vi "Alpha4.vi"() -> ()   [LabVIEW 2011]
uses:
  <vilib>/vision/NI_Vision_Development_Module.lvlib
panel:
  in  "Threshold Slider":cluster{u8, u8}(slide)={0, 6} scale=0.0..255.0
  in  "Threshold selectoin":bool
  out "Image Enhanced":T1(plugin-control)
  in  "Gamma":sgl(slide)=2.14 scale=0.0..10.0
  in  "Contrast":u8(slide)=60 scale=0.0..255.0
  in  "Brightness":u8(slide)=118 scale=0.0..255.0
  in  "Basic Morphology Operatoin":T2(ring)
  out "Threshold":T1(plugin-control)
  in  "Stop":bool
  in  "Browse":bool
  out "Original Image":T1(plugin-control)
  out "Path to Image":path
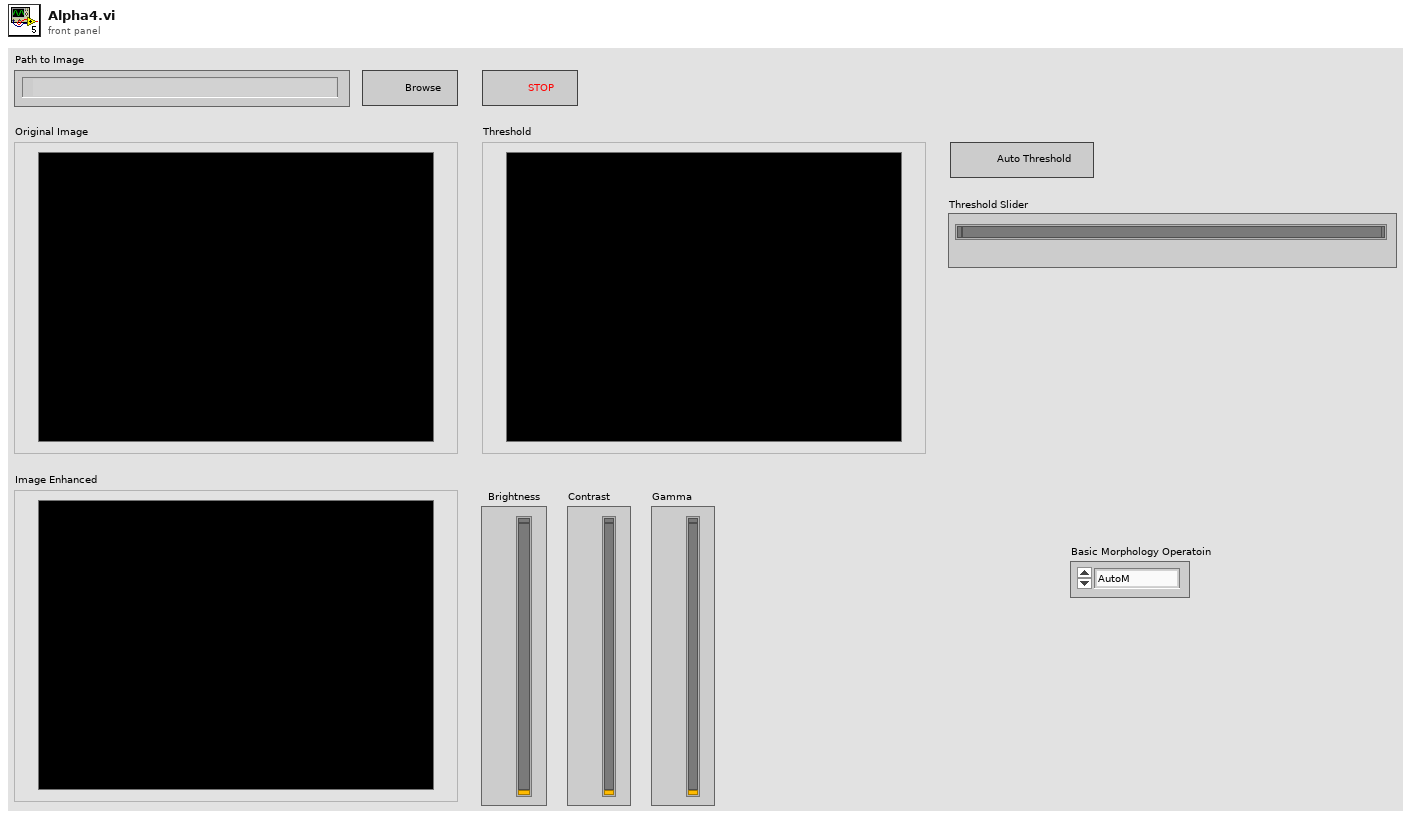
[diagram p1: front panel]
types:
  T1 = typedef "IMAQ Image.ctl" = refnum<image>
  T2 = enum16{"AutoM", "Close", "Dilate", "Erode", "Gradient", "Gradient out", "Gradient in", "Hit miss", "Open", "PClose", "POpen", "Thick", "Thin"}
  T3 = typedef "Image Type" = u32
  T4 = enum8{"Enabled", "Disabled", "Disabled and Grayed Out"}
  T5 = cluster{"Brightness":u8, "Contrast":u8, "Gamma":sgl}
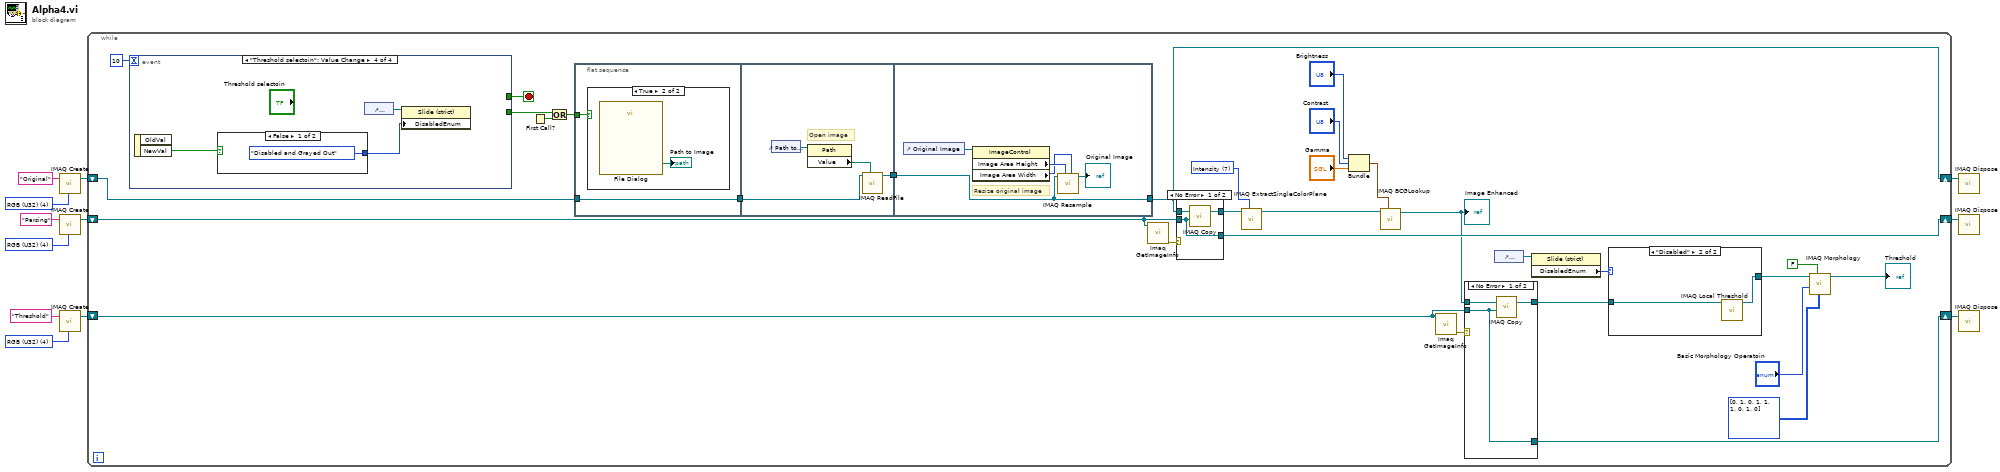
[diagram p0: block diagram]
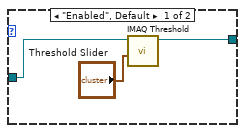
[diagram p2: hidden frame]
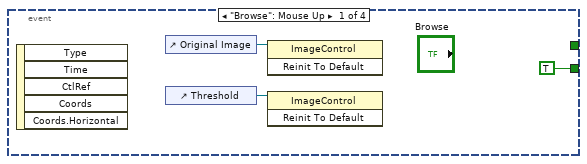
[diagram p6: hidden frame]
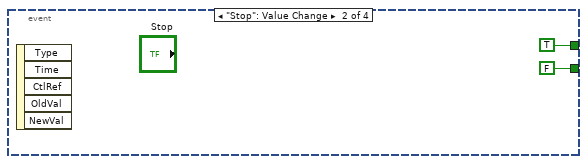
[diagram p7: hidden frame]
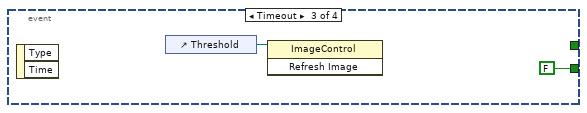
[diagram p8: hidden frame]
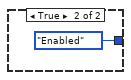
[diagram p9: hidden frame]
diagram:
  w3 = T3 4 items=["Grayscale (U8)", "Grayscale (I16)", "Grayscale (SGL)", "Complex (CSG)", "RGB (U32)", "HSL (U32)", "RGB (U64)", "Grayscale (U16)"] ("Image Type")
  w5 = T3 4 items=["Grayscale (U8)", "Grayscale (I16)", "Grayscale (SGL)", "Complex (CSG)", "RGB (U32)", "HSL (U32)", "RGB (U64)", "Grayscale (U16)"] ("Image Type")
  w8 = T3 4 items=["Grayscale (U8)", "Grayscale (I16)", "Grayscale (SGL)", "Complex (CSG)", "RGB (U32)", "HSL (U32)", "RGB (U64)", "Grayscale (U16)"] ("Image Type")
  n1 = call "IMAQ Create"("Image Name"="Original", "Image Type"=w8) -> ("New Image"=w11:T1)  [unwired: 3 in, 1 out]
  n2 = call "IMAQ Create"("Image Name"="Parsing", "Image Type"=w5) -> ("New Image"=w9:T1)  [unwired: 3 in, 1 out]
  n3 = call "IMAQ Create"("Image Name"="Threshold", "Image Type"=w3) -> ("New Image"=w2:T1)  [unwired: 3 in, 1 out]
  n4 = while {
    shift-right: [w40] -> w7
    shift-left: w11 -> [w35]
    shift-right: [w21] -> w6
    shift-left: w9 -> [w39]
    shift-right: [w18] -> w1
    shift-left: w2 -> [w19]
    stop <- w41 stop-if-true
    w26 = 7 items=["Red", "Green", "Blue", "Hue", "Saturation", "Luminance", "Value", "Intensity"] ("Color Plane")
    n5 = event shown="[3] \"Threshold selectoin\": Value Change" {
      selector: _ -> [_ _ _ _]
      dyn-events: _ -> [_ _ _ _]
      timeout: 10 -> [_ _ _ _]
      tunnel: [_ TRUE _ _] -> w41
      tunnel: [TRUE FALSE FALSE _] -> w38
      event "Browse": Mouse Up {
        n6 = event-data() -> ()  [unwired: 1 in, 5 out]
        n7 = control-ref of="Original Image"() -> (w72:refnum<vi>)
        n8 = control-ref of="Threshold"() -> (w73:refnum<vi>)
        n9 = invoke class="ImageControl" method="Reinit To Default"(reference=w72) -> ()  [unwired: 2 in, 3 out]
        n10 = invoke class="ImageControl" method="Reinit To Default"(reference=w73) -> ()  [unwired: 2 in, 3 out]
      }
      event "Stop": Value Change {
        n11 = event-data() -> ()  [unwired: 1 in, 5 out]
      }
      event Timeout {
        n12 = event-data() -> ()  [unwired: 1 in, 2 out]
        n13 = control-ref of="Threshold"() -> (w77:refnum<vi>)
        n14 = invoke class="ImageControl" method="Refresh Image"(reference=w77) -> ()  [unwired: 2 in, 3 out]
      }
      event "Threshold selectoin": Value Change {
        n15 = event-data() -> ("NewVal"=w79:bool)  [unwired: 1 in, 1 out]
        n16 = case shown="False" w79 {
          tunnel: [T4."Disabled and Grayed Out" ("Disabled") T4."Enabled" ("Disabled")] -> w80
          frame False {
          }
          frame True {
          }
        }
        n17 = control-ref of="Threshold Slider"() -> (w78:refnum<vi>)
        n18 = property class="Slide (strict)"(reference=w78, "DisabledEnum"=w80) -> ()  [unwired: 1 in, 2 out]
      }
    }
    n19 = First Call?() -> (First Call?: T/F=w37:bool)
    n20 = Or(x=w38, y=w37) -> (x .or. y?=w36:bool)
    n21 = flat-sequence {
      tunnel: w36 -> [w60]
      tunnel: w35 -> [w59]
      tunnel: [w59] -> w34
      tunnel: [w65] -> w43
      tunnel: w34 -> [w62]
      tunnel: w43 -> [w66]
      tunnel: [w66] -> w40
      frame #0 {
        n22 = case shown="True" w60 {
          frame False {
          }
          frame True {
            n23 = call "File Dialog"() -> ("selected path"=→"Path to Image":path)  [unwired: 12 in, 3 out]
          }
        }
      }
      frame #1 {
        # "Open image"
        n24 = control-ref of="Path to Image"() -> (w64:refnum<vi>)
        n25 = property class="Path"(reference=w64) -> ("Value"=w63:path)  [unwired: 1 in, 2 out]
        n26 = call "IMAQ ReadFile"("File Path"=w63, "Image"=w62) -> ("Image Out"=w65:T1)  [unwired: 5 in, 4 out]
      }
      frame #2 {
        # "Resize original image"
        n27 = control-ref of="Original Image"() -> (w70:refnum<vi>)
        n28 = property class="ImageControl"(reference=w70) -> ("Image Area Height"=w69:u32, "Image Area Width"=w68:u32)  [unwired: 1 in, 2 out]
        n29 = call "IMAQ Resample"("X Resolution"=w68, "Y Resolution"=w69, "Image Src"=w66) -> ("Image Dst Out"=→"Original Image":T1)  [unwired: 7 in, 1 out]
      }
    }
    n30 = call "Imaq GetImageInfo"("Image"=w39) -> ("error out"=w42:errorcluster)  [unwired: 1 in, 9 out]
    n31 = case shown="No Error" w42 {
      tunnel: w39 -> [w54 w57]
      tunnel: w40 -> [w56 w58]
      tunnel: [w55 w58] -> w22
      tunnel: [w54 w57] -> w21
      frame No Error {
        n32 = call "IMAQ Copy"("Image Dst"=w54, "Image Src"=w56) -> ("Image Dst Out"=w55:T1)  [unwired: 4 in, 1 out]
      }
      frame Error {
      }
    }
    n33 = call "IMAQ ExtractSingleColorPlane"("Color Plane"=w26, "Image Src"=w22) -> ("Image Dst Out"=w27:T1)  [unwired: 2 in, 7 out]
    n34 = Bundle("Brightness"="Brightness", "Contrast"="Contrast", "Gamma"="Gamma") -> (w25:T5)  [unwired: 1 in]
    n35 = call "IMAQ BCGLookup"("Image Src"=w27, "BCG Values"=w25) -> ("Image Dst Out"=w17:T1)  [unwired: 3 in, 3 out]
    "Image Enhanced" <- w17
    n36 = call "Imaq GetImageInfo"("Image"=w19) -> ("error out"=w20:errorcluster)  [unwired: 1 in, 9 out]
    n37 = case shown="No Error" w20 {
      tunnel: w19 -> [w49 w52]
      tunnel: w17 -> [w51 w53]
      tunnel: [w50 w53] -> w13
      tunnel: [w49 w52] -> w18
      frame No Error {
        n38 = call "IMAQ Copy"("Image Dst"=w49, "Image Src"=w51) -> ("Image Dst Out"=w50:T1)  [unwired: 4 in, 1 out]
      }
      frame Error {
      }
    }
    n39 = control-ref of="Threshold Slider"() -> (w14:refnum<vi>)
    n40 = property class="Slide (strict)"(reference=w14) -> ("DisabledEnum"=w16:T4)  [unwired: 1 in, 2 out]
    n41 = case shown="\"Disabled\"" w16 {
      tunnel: [w45 w48] -> w15
      tunnel: w13 -> [w44 w47]
      frame "Enabled", Default {
        n42 = call "IMAQ Threshold"("Range"="Threshold Slider", "Image Src"=w44) -> ("Image Dst Out"=w45:T1)  [unwired: 4 in, 5 out]
      }
      frame "Disabled" {
        n43 = call "IMAQ Local Threshold"("Image Src"=w47) -> ("Image Dst Out"=w48:T1)  [unwired: 13 in, 1 out]
      }
    }
    n44 = call "IMAQ Morphology"("Structuring Element"=i32[][] [[0, 1, 0], [1, 1, 1], [0, 1, 0]], "Square/Hexa (Square)"=FALSE, "Operation"="Basic Morphology Operatoin", "Image Src"=w15) -> ("Image Dst Out"=→"Threshold":T1)  [unwired: 3 in, 4 out]
  }
  n45 = call "IMAQ Dispose"("Image"=w7) -> ()  [unwired: 5 in, 1 out]
  n46 = call "IMAQ Dispose"("Image"=w6) -> ()  [unwired: 5 in, 1 out]
  n47 = call "IMAQ Dispose"("Image"=w1) -> ()  [unwired: 5 in, 1 out]
